vi "EEPROM Read-Write, single slot, standalone.vi"() -> ()   [LabVIEW 2015]
uses:
  Ctls/EEPROM page.ctl
panel:
  out "Power off ACK":bool
  out "Power on ACK":bool
  out "Single slot EEPROM values returned":T1[](array[typedef])
  in  "Slot":u8 max=7
  in  "Single slot EEPROM values":T1[](array[typedef])=[{"Pmin (Pa)"=0.0, "Pmax (Pa)"=0.0, "maxCount"=0, "minCount"=0, "Poffset (Pa)"=0.0}, {"Pmin (Pa)"=0.0, "Pmax (Pa)"=0.0, "maxCount"=0, "minCount"=0, "Poffset (Pa)"=0.0}, {"Pmin (Pa)"=0.0, "Pmax (Pa)"=0.0, "maxCount"=0, "minCount"=0, "Poffset (Pa)"=0.0}, {"Pmin (Pa)"=0.0, "Pmax (Pa)"=0.0, "maxCount"=0, "minCount"=0, "Poffset (Pa)"=0.0}, {"Pmin (Pa)"=0.0, "Pmax (Pa)"=0.0, "maxCount"=0, "minCount"=0, "Poffset (Pa)"=0.0}, {"Pmin (Pa)"=0.0, "Pmax (Pa)"=0.0, "maxCount"=0, "minCount"=0, "Poffset (Pa)"=0.0}, {"Pmin (Pa)"=0.0, "Pmax (Pa)"=0.0, "maxCount"=0, "minCount"=0, "Poffset (Pa)"=0.0}, {"Pmin (Pa)"=0.0, "Pmax (Pa)"=0.0, "maxCount"=0, "minCount"=0, "Poffset (Pa)"=0.0}]
  out "Data ACK":bool
  in  "VISA resource name in":refnum<visa-resource-name>
  out "Error out":errorcluster
  in  "R / W":string(combo)="R"
  # "0"
  # "1"
  # "2"
  # "3"
  # "4"
  # "5"
  # "6"
  # "7"
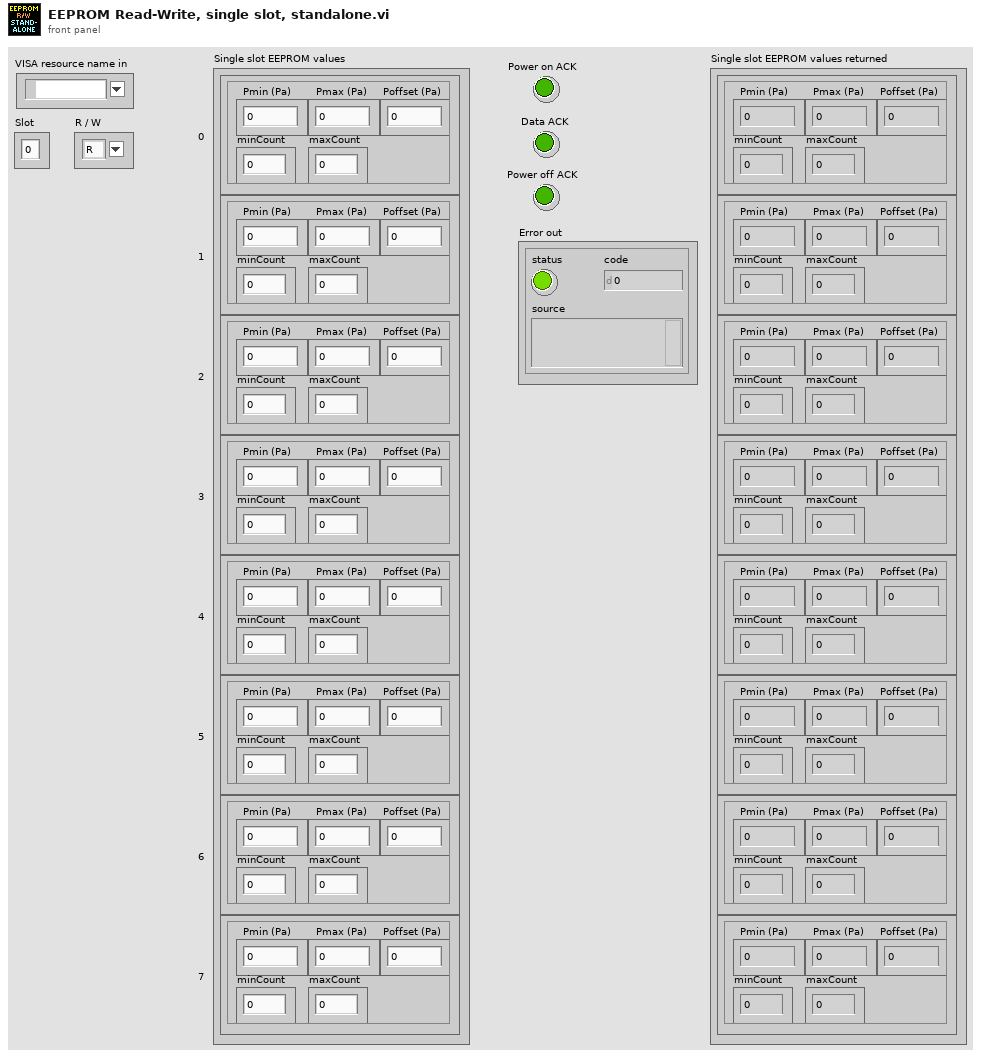
[diagram p1: front panel]
types:
  T1 = typedef "EEPROM page.ctl" = cluster{"Pmin (Pa)":sgl, "Pmax (Pa)":sgl, "maxCount":u16, "minCount":u16, "Poffset (Pa)":sgl}
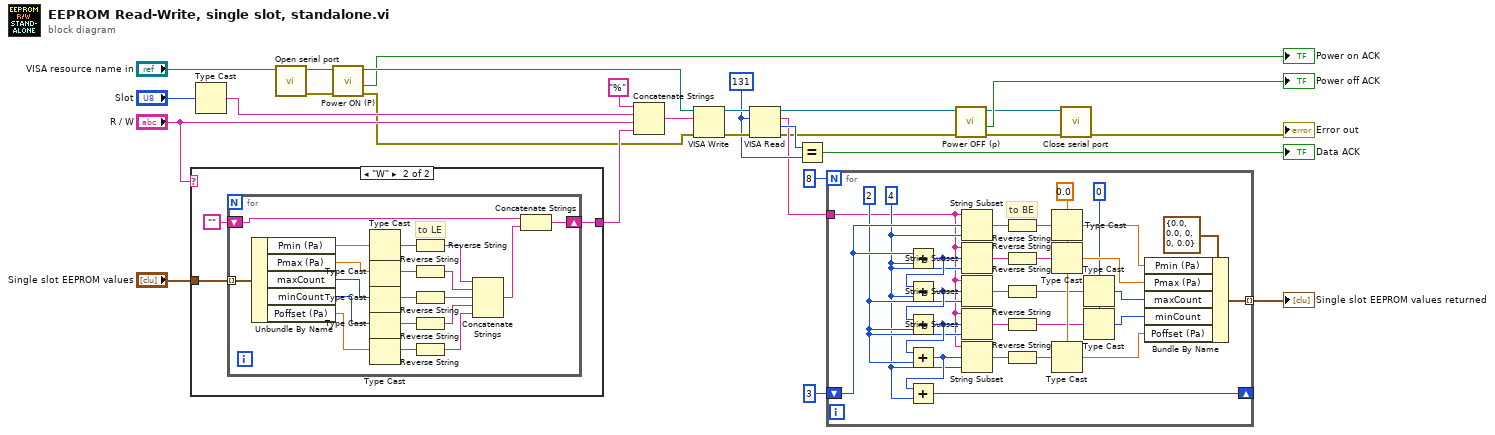
[diagram p0: block diagram]
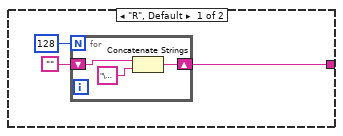
[diagram p2: hidden frame]
diagram:
  w22 = u32 131 ("byte count")
  n1 = case shown="\"W\"" "R / W" {
    tunnel: "Single slot EEPROM values" -> [_ w37]
    tunnel: [w30 w35] -> w19
    frame "R", Default {
      n2 = for {
        N: 128 -> [_]
        shift-right: [w33] -> w30
        shift-left: "" -> [w32]
        n3 = Concatenate Strings(w32, "\u0000") -> (w33:string)
      }
    }
    frame "W" {
      n4 = for {
        tunnel: w37 -> [w56] mode=indexing
        shift-right: [w39] -> w35
        shift-left: "" -> [w38]
        # "to LE"
        n5 = Unbundle By Name(w56) -> ("Pmin (Pa)"=w55:sgl, "Pmax (Pa)"=w49:sgl, "maxCount"=w48:u16, "minCount"=w47:u16, "Poffset (Pa)"=w46:sgl)
        n6 = Type Cast(x=w55) -> (*(type *) &x=w54:string)  [unwired: 1 in]
        n7 = Type Cast(x=w49) -> (*(type *) &x=w53:string)  [unwired: 1 in]
        n8 = Type Cast(x=w48) -> (*(type *) &x=w52:string)  [unwired: 1 in]
        n9 = Type Cast(x=w47) -> (*(type *) &x=w51:string)  [unwired: 1 in]
        n10 = Type Cast(x=w46) -> (*(type *) &x=w50:string)  [unwired: 1 in]
        n11 = Reverse String(1:w54) -> (0:w45:string)
        n12 = Reverse String(1:w53) -> (0:w44:string)
        n13 = Reverse String(1:w52) -> (0:w43:string)
        n14 = Reverse String(1:w51) -> (0:w42:string)
        n15 = Reverse String(1:w50) -> (0:w41:string)
        n16 = Concatenate Strings(w45, w44, w43, w42, w41) -> (w40:string)
        n17 = Concatenate Strings(w38, w40) -> (w39:string)
      }
    }
  }
  n18 = Type Cast(x="Slot") -> (*(type *) &x=w17:string)  [unwired: 1 in]
  n19 = call "Open serial port.vi"("VISA resource name"="VISA resource name in") -> ("Error out"=w1:errorcluster, "VISA resource name out"=w2:refnum<visa-resource-name>)  [unwired: 9 in]
  n20 = call "Power ON (P).vi"("Error In"=w1, "VISA resource name in"=w2) -> ("Error out"=w8:errorcluster, "ACK"=→"Power on ACK":bool, "VISA resource name out"=w11:refnum<visa-resource-name>)  [unwired: 7 in]
  n21 = Concatenate Strings("%" ("string"), w17, "R / W", w19) -> (w24:string)
  n22 = VISA Write(VISA resource name=w11, write buffer=w24, error in (no error)=w8) -> (VISA resource name out=w27:refnum<visa-resource-name>, error out=w26:errorcluster)  [unwired: 1 out]
  n23 = VISA Read(VISA resource name=w27, byte count=w22, error in (no error)=w26) -> (VISA resource name out=w9:refnum<visa-resource-name>, read buffer=w12:string, return count=w23:u32, error out=w7:errorcluster)
  n24 = Equal?(x=w23, y=w22) -> (x = y?=→"Data ACK":bool)
  n25 = for {
    N: 8 -> [_]
    shift-right: [w76] -> _
    shift-left: 3 ("offset (0)") -> [w83]
    tunnel: [w68] -> w14 mode=indexing
    tunnel: w12 -> [w67]
    w79 = 2 ("length (rest)")
    w77 = 4 ("length (rest)")
    w71 = u16 0
    w84 = sgl 0.0
    # "to BE"
    n26 = Add(x=w83, y=w77) -> (x+y=w82:i32)
    n27 = Add(x=w82, y=w77) -> (x+y=w81:i32)
    n28 = Add(x=w81, y=w79) -> (x+y=w80:i32)
    n29 = Add(x=w80, y=w79) -> (x+y=w78:i32)
    n30 = Add(x=w78, y=w77) -> (x+y=w76:i32)
    n31 = String Subset(string=w67, offset (0)=w83, length (rest)=w77) -> (substring=w66:string)
    n32 = String Subset(string=w67, offset (0)=w82, length (rest)=w77) -> (substring=w64:string)
    n33 = String Subset(string=w67, offset (0)=w81, length (rest)=w79) -> (substring=w62:string)
    n34 = String Subset(string=w67, offset (0)=w80, length (rest)=w79) -> (substring=w60:string)
    n35 = String Subset(string=w67, offset (0)=w78, length (rest)=w77) -> (substring=w58:string)
    n36 = Reverse String(1:w66) -> (0:w65:string)
    n37 = Reverse String(1:w64) -> (0:w63:string)
    n38 = Reverse String(1:w62) -> (0:w61:string)
    n39 = Reverse String(1:w60) -> (0:w59:string)
    n40 = Reverse String(1:w58) -> (0:w57:string)
    n41 = Type Cast(type=w84, x=w65) -> (*(type *) &x=w74:sgl)
    n42 = Type Cast(type=w84, x=w63) -> (*(type *) &x=w73:sgl)
    n43 = Type Cast(type=w84, x=w57) -> (*(type *) &x=w69:sgl)
    n44 = Type Cast(type=w71, x=w61) -> (*(type *) &x=w72:u16)
    n45 = Type Cast(type=w71, x=w59) -> (*(type *) &x=w70:u16)
    n46 = Bundle By Name(cluster=T1 {"Pmin (Pa)"=0.0, "Pmax (Pa)"=0.0, "maxCount"=0, "minCount"=0, "Poffset (Pa)"=0.0} ("Page"), "Pmin (Pa)"=w74, "Pmax (Pa)"=w73, "maxCount"=w72, "minCount"=w70, "Poffset (Pa)"=w69) -> (w68:T1)
  }
  "Single slot EEPROM values returned" <- w14
  n47 = call "Power OFF (p).vi"("Error In"=w7, "VISA resource name in"=w9) -> ("Error out"=w4:errorcluster, "ACK"=→"Power off ACK":bool, "VISA resource name out"=w5:refnum<visa-resource-name>)  [unwired: 7 in]
  n48 = call "Close serial port.vi"("Error in"=w4, "VISA resource name"=w5) -> ("Error out"=→"Error out":errorcluster)  [unwired: 9 in]
